vi "Configure Connection Dialog.vi"(8 "error in (no error)":errorcluster, 10 "Current Connection":T8, 11 "Channel Editor State":T1={"Modules and Connections"=[{" Module Path"="", "Short Module Path"="", "Product Name"="", "Possible Connections"=[]}, {" Module Path"="", "Short Module Path"="", "Product Name"="", "Possible Connections"=[]}], "Alias Mappings UI"=[], "Mappings by Module UI"=[]}) -> (0 "error out":errorcluster, 1 "Connection (R,S,D)":T7, 2 "Canceled?":bool)   [LabVIEW 2017, in "Routing and Faulting System Explorer.lvlib"]
uses:
  Routing and Faulting System Explorer.lvlib
  Connection Row.ctl
  Shared/Connection.ctl
  Channel Editor State.ctl
  Possible Connections.ctl
  Shared/Routing and Faulting Hardware API/Types/Possible Connections for Endpoint.ctl
  Shared/Alias Mapping.ctl
  Shared/Alias Endpoint.ctl
  Alias Map by Module.ctl
  <vilib>/event_ctls.llb/lveventtype.ctl
  Shared/Constants.vi
  Shared/Routing and Faulting Shared.lvlib
  Shared/Routing and Faulting Hardware API/Routing and Faulting Hardware API.lvlib
panel:
  out "Product Name List":string[](array[string])
  out "Module Index":i32
  out "Initial Module":string
  out "Initial Destination":string
  out "Initial Source":string
  in  "Module":string(combo)
  in  "Cancel Button":bool
  in  "OK Button":bool
  in  "Destination":string(combo)
  in  "Source":string(combo)
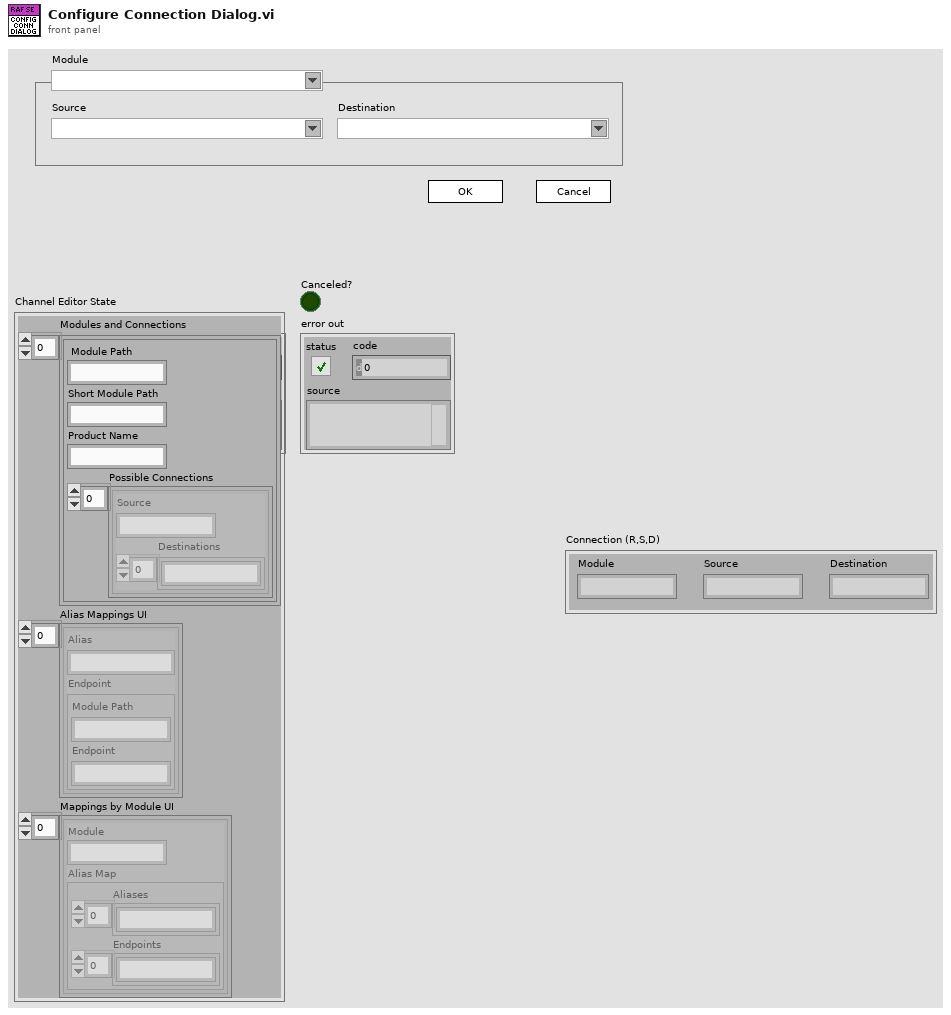
[diagram p1: front panel]
types:
  T1 = typedef "Routing and Faulting System Explorer.lvlib/Channel Editor State.ctl" = cluster{"Modules and Connections":T2[], "Alias Mappings UI":T4[], "Mappings by Module UI":T6[]}
  T2 = typedef "Routing and Faulting System Explorer.lvlib/Possible Connections.ctl" = cluster{" Module Path":string, "Short Module Path":string, "Product Name":string, "Possible Connections":T3[]}
  T3 = typedef "Routing and Faulting Hardware API.lvlib/Possible Connections for Endpoint.ctl" = cluster{"Source":string, "Destinations":string[]}
  T4 = typedef "Routing and Faulting Shared.lvlib/Alias Mapping.ctl" = cluster{"Alias":string, "Endpoint":T5}
  T5 = typedef "Routing and Faulting Shared.lvlib/Alias Endpoint.ctl" = cluster{"Module Path":string, "Endpoint":string}
  T6 = typedef "Routing and Faulting System Explorer.lvlib/Alias Map by Module.ctl" = cluster{"Module":string, "Alias Map":cluster{"Aliases":string[], "Endpoints":string[]}}
  T7 = typedef "Routing and Faulting Shared.lvlib/Connection.ctl" = cluster{"Module":string, "Source":string, "Destination":string}
  T8 = typedef "Routing and Faulting System Explorer.lvlib/Connection Row.ctl" = cluster{"Source":string, "Destination":string, "Edit":bool, "Remove":bool}
  T9 = typedef "lveventtype.ctl" = enum32{"Null", "Timeout", "Annotation Menu Selection", "Annotation Menu Selection?", "App Instance Close", "App Instance Close?", "Autoscale Range Change", "Bookmark Info Change", "Cell Edit", "Cell Edit?", "Cursor Grab", "Cursor Grab?", "Cursor Menu Selection", "Cursor Menu Selection?", "Cursor Move", "Cursor Release", "Data Change", "Direction Change", "Display State Change", "Drag Ended", "Drag Enter", "Drag Leave", "Drag Over", "Drag Source Update", "Drag Starting", "Drag Starting?", "Drop", "Exec State Change", "Key Down", "Key Down?", "Key Repeat", "Key Repeat?", "Key Up", "Listbox Double Click", "Menu Activation?", "Menu Selection (App)", "Menu Selection? (App)", "Menu Selection (User)", "Mouse Down", "Mouse Down?", "Mouse Enter", "Mouse Leave", "Mouse Move", "Mouse Up", "Mouse Wheel", "NI Security User Change (App)", "Pane Size", "Panel Close", "Panel Close?", "Panel Resize", "Plot Attribute Change", "Scale Range Change", "Shortcut Menu Activation?", "Shortcut Menu Selection (App)", "Shortcut Menu Selection? (App)", "Shortcut Menu Selection (User)", "Tree Double Click", "Tree Drag", "Tree Drag?", "Tree Drop", "Tree Drop?", "Tree Item Close", "Tree Item Close?", "Tree Item Open", "Tree Item Open?", "User Event", "Value Change"}
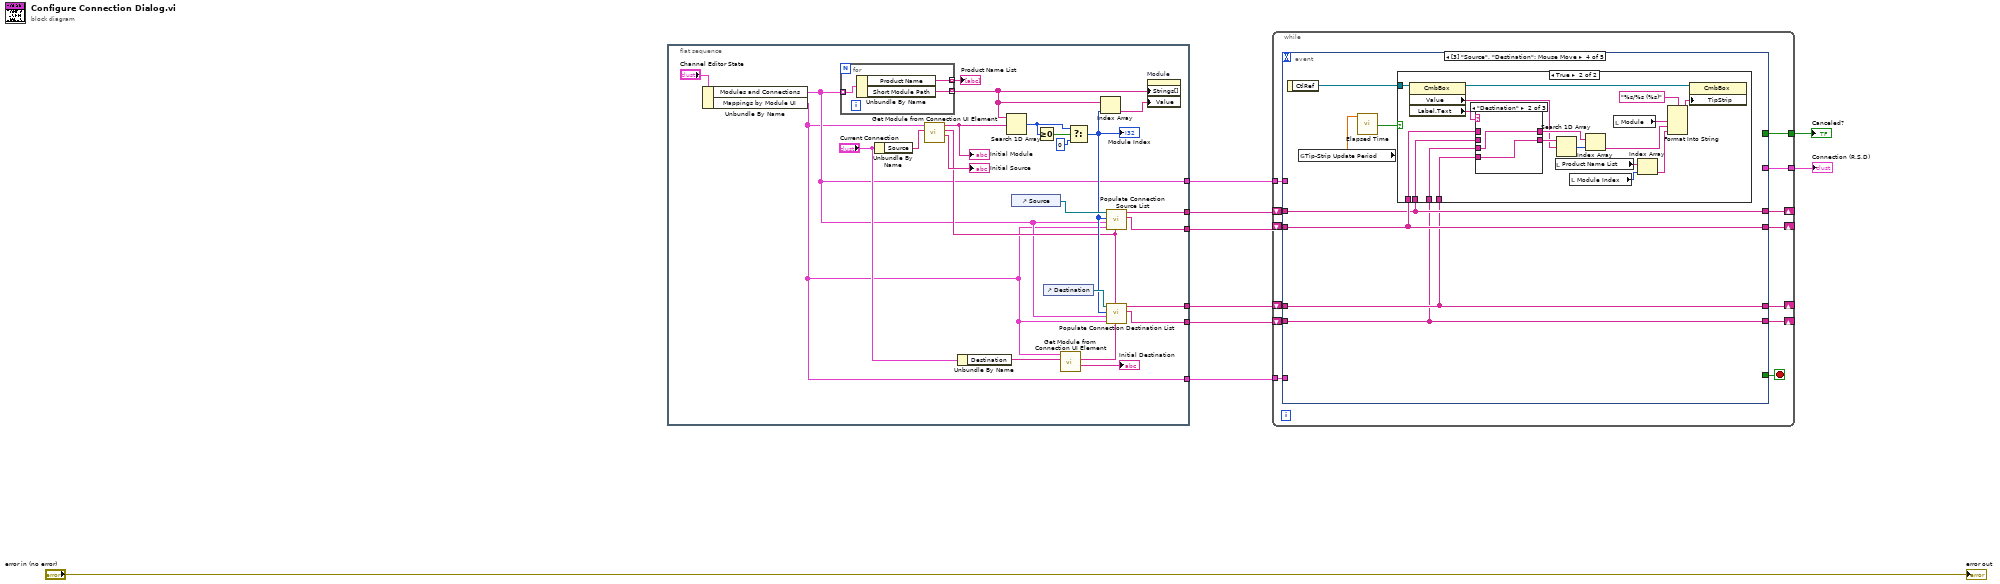
[diagram p0: block diagram]
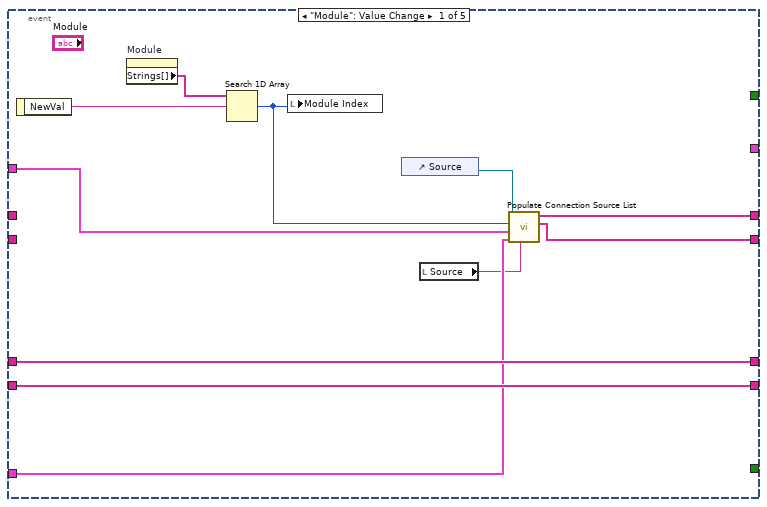
[diagram p2: hidden frame]
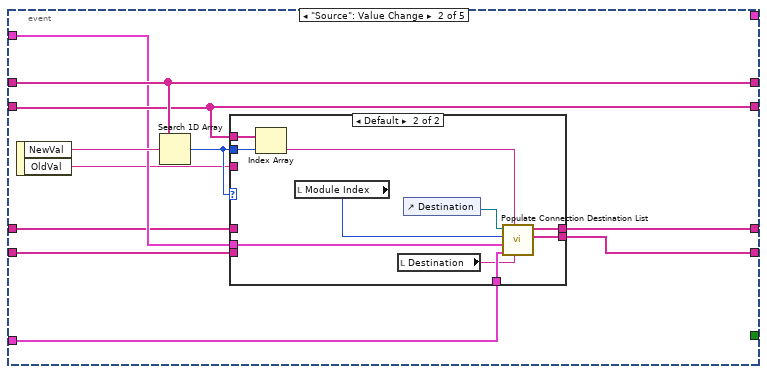
[diagram p3: hidden frame]
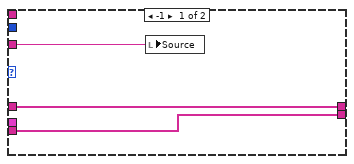
[diagram p4: hidden frame]
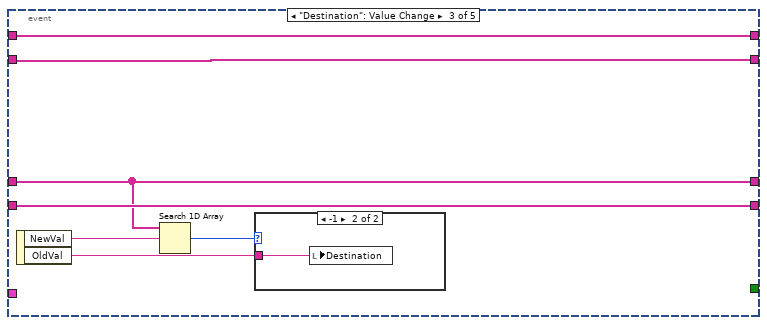
[diagram p5: hidden frame]
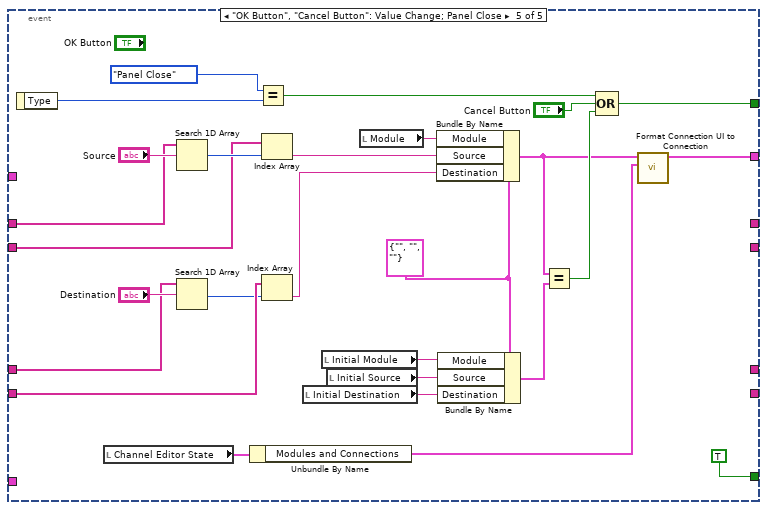
[diagram p10: hidden frame]
diagram:
  n1 = flat-sequence {
    tunnel: [w29] -> w7
    tunnel: [w11] -> w2
    tunnel: [w26] -> w6
    tunnel: [w25] -> w5
    tunnel: [w12] -> w4
    tunnel: [w28] -> w3
    frame #0 {
      n2 = Unbundle By Name("Channel Editor State") -> ("Modules and Connections"=w12:T2[], "Mappings by Module UI"=w11:T6[])
      n3 = for {
        tunnel: w12 -> [w36] mode=indexing
        tunnel: [w35] -> w33 mode=indexing
        tunnel: [w34] -> w10 mode=indexing
        n4 = Unbundle By Name(w36) -> ("Product Name"=w34:string, "Short Module Path"=w35:string)
      }
      "Product Name List" <- w10
      n5 = Unbundle By Name("Current Connection") -> ("Source"=w19:string)
      n6 = call "Get Module from Connection UI Element.vi"("Alias or Full Endpoint"=w19, "Alias Mappings by Module"=w11) -> ("Long Endpoint"=→"Initial Source":string, "Short Endpoint"=w17:string, "Module"=w31:string)  [unwired: 7 in]
      "Initial Module" <- w31
      n7 = Unbundle By Name("Current Connection") -> ("Destination"=w16:string)
      n8 = Search 1D Array(1D array=w33, element=w31) -> (index of element=w23:i32)  [unwired: 1 in]
      n9 = control-ref of="Source"() -> (w30:refnum<vi>)
      n10 = Greater Or Equal To 0?(x=w23) -> (x >= 0?=w24:bool)
      n11 = control-ref of="Destination"() -> (w27:refnum<vi>)
      n12 = call "Get Module from Connection UI Element.vi"("Alias or Full Endpoint"=w16, "Alias Mappings by Module"=w11) -> ("Long Endpoint"=→"Initial Destination":string, "Short Endpoint"=w14:string)  [unwired: 7 in, 1 out]
      n13 = Select(t=w23, s=w24, f=0) -> (s? t:f=w20:i32)
      "Module Index" <- w20
      n14 = Index Array(array=w33, index=w20) -> (element=w32:string)
      n15 = call "Populate Connection Source List.vi"("initial Source"=w17, "Alias Mappings by Module"=w11, "Possible Connections"=w12, "Module Index"=w20, "Source Reference"=w30) -> ("Endpoint List"=w28:string[], "Alias List"=w29:string[])  [unwired: 5 in]
      n16 = call "Populate Connection Destination List.vi"("initial Destination"=w14, "Source"=w17, "Alias Mappings by Module"=w11, "Possible Connections"=w12, "Module Index"=w20, "Destination Reference"=w27) -> ("Endpoint List"=w25:string[], "Alias List"=w26:string[])  [unwired: 4 in]
      n17 = property on="Module" class="CmbBox"("Strings[]"=w33, "Value"=w32) -> ()  [unwired: 2 in, 2 out]
    }
  }
  n18 = while {
    tunnel: [w48] -> w9
    tunnel: w4 -> [w47]
    shift-right: [w43] -> _
    shift-left: w7 -> [w46]
    shift-right: [w42] -> _
    shift-left: w3 -> [w45]
    tunnel: w2 -> [w44]
    shift-right: [w41] -> _
    shift-left: w6 -> [w39]
    shift-right: [w40] -> _
    shift-left: w5 -> [w38]
    tunnel: [w37] -> w1
    stop <- w49 stop-if-true
    n19 = event shown="[3] \"Source\", \"Destination\": Mouse Move" {
      selector: _ -> [_ _ _ _ _]
      dyn-events: _ -> [_ _ _ _ _]
      timeout: _ -> [_ _ _ _ _]
      tunnel: [_ _ _ _ TRUE] -> w49
      tunnel: [_ _ _ _ w144] -> w48
      tunnel: w47 -> [w53 w66 _ _ _]
      tunnel: w46 -> [_ w70 w90 w98 w140]
      tunnel: w45 -> [_ w67 w89 w99 w139]
      tunnel: w44 -> [w54 w65 _ _ _]
      tunnel: [w59 w70 w90 w98 _] -> w43
      tunnel: [w58 w67 w89 w99 _] -> w42
      tunnel: [w57 w69 w87 w97 _] -> w41
      tunnel: [w56 w68 w88 w96 _] -> w40
      tunnel: w39 -> [w57 w63 w87 w97 w136]
      tunnel: w38 -> [w56 w62 w88 w96 w135]
      tunnel: [_ _ _ _ w122] -> w37
      event "Module": Value Change {
        n20 = event-data() -> ("NewVal"=w60:string)  [unwired: 1 in]
        n21 = property on="Module" class="CmbBox"() -> ("Strings[]"=w52:string[])  [unwired: 2 in, 2 out]
        n22 = Search 1D Array(1D array=w52, element=w60) -> (index of element=w51:i32)  [unwired: 1 in]
        n23 = local write "Module Index"(w51) -> ()
        n24 = control-ref of="Source"() -> (w55:refnum<vi>)
        n25 = local read "Source"() -> (w50:string)
        n26 = call "Populate Connection Source List.vi"("initial Source"=w50, "Alias Mappings by Module"=w54, "Possible Connections"=w53, "Module Index"=w51, "Source Reference"=w55) -> ("Endpoint List"=w58:string[], "Alias List"=w59:string[])  [unwired: 5 in]
      }
      event "Source": Value Change {
        n27 = event-data() -> ("NewVal"=w71:string, "OldVal"=w61:string)  [unwired: 1 in]
        n28 = Search 1D Array(1D array=w70, element=w71) -> (index of element=w64:i32)  [unwired: 1 in]
        n29 = case shown="Default" w64 {
          tunnel: w64 -> [_ w84]
          tunnel: [w74 w83] -> w69
          tunnel: [w73 w82] -> w68
          tunnel: w67 -> [_ w81]
          tunnel: w66 -> [_ w79]
          tunnel: w65 -> [_ w77]
          tunnel: w63 -> [w74 _]
          tunnel: w62 -> [w73 _]
          tunnel: w61 -> [w72 _]
          frame -1 {
            n30 = local write "Source"(w72) -> ()
          }
          frame Default {
            n31 = Index Array(array=w81, index=w84) -> (element=w76:string)
            n32 = local read "Module Index"() -> (w80:i32)
            n33 = local read "Destination"() -> (w75:string)
            n34 = control-ref of="Destination"() -> (w78:refnum<vi>)
            n35 = call "Populate Connection Destination List.vi"("initial Destination"=w75, "Source"=w76, "Alias Mappings by Module"=w77, "Possible Connections"=w79, "Module Index"=w80, "Destination Reference"=w78) -> ("Endpoint List"=w82:string[], "Alias List"=w83:string[])  [unwired: 4 in]
          }
        }
      }
      event "Destination": Value Change {
        n36 = event-data() -> ("NewVal"=w91:string, "OldVal"=w85:string)  [unwired: 1 in]
        n37 = Search 1D Array(1D array=w87, element=w91) -> (index of element=w86:i32)  [unwired: 1 in]
        n38 = case shown="-1" w86 {
          tunnel: w85 -> [_ w92]
          frame Default {
          }
          frame -1 {
            n39 = local write "Destination"(w92) -> ()
          }
        }
      }
      event "Source", "Destination": Mouse Move {
        n40 = event-data() -> ("CtlRef"=w95:refnum<vi>)  [unwired: 1 in]
        n41 = global read "Constants.vi" "Tip-Strip Update Period"() -> (w94:dbl)
        n42 = call "Elapsed Time"("Time Target (s)"=w94) -> ("Time has Elapsed"=w93:bool)  [unwired: 11 in, 7 out]
        n43 = case shown="True" w93 {
          tunnel: w99 -> [_ w109]
          tunnel: w98 -> [_ w108]
          tunnel: w97 -> [_ w107]
          tunnel: w96 -> [_ w106]
          tunnel: w95 -> [_ w102]
          frame False {
            # "Only process mouse moves every 10ms"
          }
          frame True {
            n44 = property class="CmbBox"(reference=w102) -> (reference out=w101:refnum<vi>, "Value"=w100:string, "Label.Text"=w103:string)  [unwired: 1 in, 1 out]
            n45 = case shown="\"Destination\"" w103 {
              tunnel: w109 -> [w118 _ _]
              tunnel: w108 -> [w119 _ _]
              tunnel: w107 -> [_ w121 _]
              tunnel: w106 -> [_ w120 _]
              tunnel: [w119 w121 _] -> w105
              tunnel: [w118 w120 _] -> w104
              frame "Source" {
              }
              frame "Destination" {
              }
              frame Default {
              }
            }
            n46 = local read "Product Name List"() -> (w113:string[])
            n47 = Search 1D Array(1D array=w105, element=w100) -> (index of element=w117:i32)  [unwired: 1 in]
            n48 = local read "Module Index"() -> (w112:i32)
            n49 = Index Array(array=w104, index=w117) -> (element=w114:string)
            n50 = local read "Module"() -> (w115:string)
            n51 = Index Array(array=w113, index=w112) -> (element=w111:string)
            n52 = Format Into String(format string="%s/%s (%s)", w115, w114, w111) -> (resulting string=w110:string)  [unwired: 2 in, 1 out]
            n53 = property class="CmbBox"(reference=w101, "TipStrip"=w110) -> ()  [unwired: 1 in, 2 out]
          }
        }
      }
      event "OK Button", "Cancel Button": Value Change; Panel Close {
        w132 = T7 {"Module"="", "Source"="", "Destination"=""} ("Connection (R,S,D)")
        n54 = event-data() -> ("Type"=w146:T9)  [unwired: 1 in]
        n55 = local read "Channel Editor State"() -> (w125:T1)
        n56 = Search 1D Array(1D array=w140, element="Source") -> (index of element=w142:i32)  [unwired: 1 in]
        n57 = Search 1D Array(1D array=w136, element="Destination") -> (index of element=w134:i32)  [unwired: 1 in]
        n58 = Unbundle By Name(w125) -> ("Modules and Connections"=w123:T2[])
        n59 = Equal?(x=lveventtype."Panel Close" ("Type"), y=w146) -> (x = y?=w127:bool)
        n60 = Index Array(array=w139, index=w142) -> (element=w138:string)
        n61 = Index Array(array=w135, index=w134) -> (element=w133:string)
        n62 = local read "Initial Destination"() -> (w128:string)
        n63 = local read "Initial Module"() -> (w130:string)
        n64 = local read "Initial Source"() -> (w129:string)
        n65 = local read "Module"() -> (w143:string)
        n66 = Bundle By Name(cluster=w132, "Module"=w143, "Source"=w138, "Destination"=w133) -> (w124:T7)
        n67 = Bundle By Name(cluster=w132, "Module"=w130, "Source"=w129, "Destination"=w128) -> (w131:T7)
        n68 = Equal?(x=w124, y=w131) -> (x = y?=w126:bool)
        n69 = Compound Arithmetic op=OR(w127, "Cancel Button", w126) -> (w144:bool)
        n70 = call "Format Connection UI to Connection.vi"("Modules and Connections"=w123, "Connection UI"=w124) -> ("Connection"=w122:T7)  [unwired: 9 in]
      }
    }
  }
  "Canceled?" <- w9
  "Connection (R,S,D)" <- w1
  "error out" <- "error in (no error)"
